vi "open select sample sheet.vi"(7 "Number of Sample Sheets":i32, 8 "error in (no error)":errorcluster, 9 "Worksheet Names":string[](array[string]), 10 "input 1":i32, 11 "NI_report in":refnum<class "NI_report.lvclass">) -> (0 "error out":errorcluster, 1 "Current Sample Sheet":string, 3 "NI_report out":refnum<class "NI_report.lvclass">)   [LabVIEW 2016]
uses:
  <vilib>/Utility/NIReport.llb/NI_report.lvclass
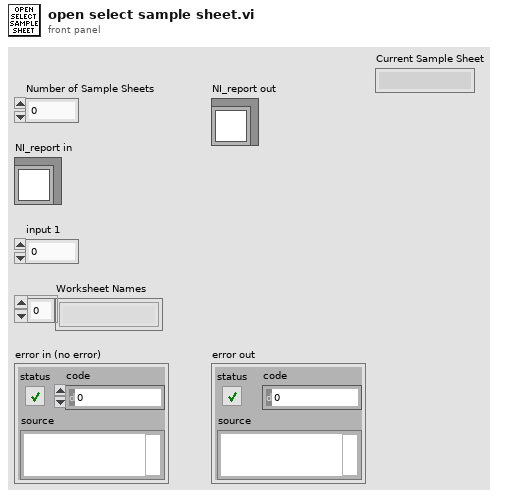
[diagram p1: front panel]
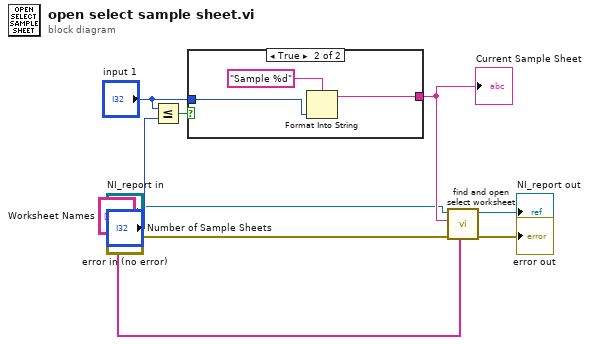
[diagram p0: block diagram]
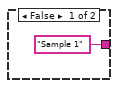
[diagram p2: hidden frame]
diagram:
  n1 = Less Or Equal?(x="input 1", y="Number of Sample Sheets") -> (x <= y?=w7:bool)
  n2 = case shown="True" w7 {
    tunnel: ["Sample 1" w13] -> w6
    tunnel: "input 1" -> [_ w12]
    frame False {
    }
    frame True {
      n3 = Format Into String(format string="Sample %d" ("Worksheet Name 1"), w12) -> (resulting string=w13:string)  [unwired: 2 in, 1 out]
    }
  }
  "Current Sample Sheet" <- w6
  n4 = call "find and open select worksheet.vi"("Worksheet Names"="Worksheet Names", "error in (no error)"="error in (no error)", "Worksheet Name in"=w6, "NI_report in"="NI_report in") -> ("error out"=→"error out":errorcluster, "NI_report out"=→"NI_report out":refnum<class "NI_report.lvclass">)  [unwired: 6 in]
